vi "Width_Height to File Name.vi"(7 "include size in file name?":bool, 8 "keyword (\"\")":string, 10 "size":T1, 11 "VI file name (no extension)":string) -> (3 "file name":string)   [LabVIEW 2010, in "NI_SE_Front Panel Layout.lvlib"]
uses:
  NI_SE_Front Panel Layout.lvlib
  <vilib>/Utility/miscctls.llb/LVPointTypeDef.ctl
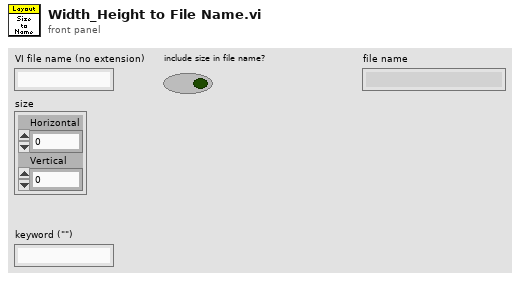
[diagram p1: front panel]
types:
  T1 = typedef "LVPointTypeDef.ctl" = cluster{"Horizontal":i16, "Vertical":i16}
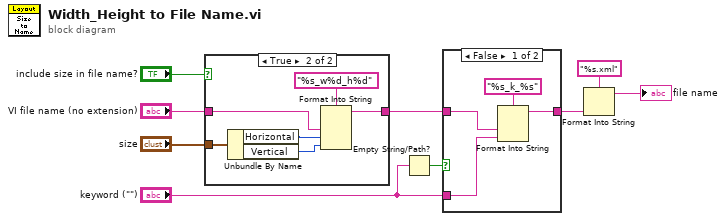
[diagram p0: block diagram]
diagram:
  n1 = case shown="True" "include size in file name?" {
    tunnel: "VI file name (no extension)" -> [w10 w15]
    tunnel: "size" -> [_ w13]
    tunnel: [w10 w14] -> w8
    frame False {
    }
    frame True {
      n2 = Unbundle By Name(w13) -> ("Horizontal"=w12:i16, "Vertical"=w11:i16)
      n3 = Format Into String(format string="%s_w%d_h%d", w15, w12, w11) -> (resulting string=w14:string)  [unwired: 2 in, 1 out]
    }
  }
  n4 = Empty String/Path?(string/path="keyword (\"\")") -> (empty?=w7:bool)
  n5 = case shown="False" w7 {
    tunnel: w8 -> [w19 w21]
    tunnel: "keyword (\"\")" -> [w17 _]
    tunnel: [w18 w21] -> w5
    frame False {
      n6 = Format Into String(format string="%s_k_%s", w19, w17) -> (resulting string=w18:string)  [unwired: 2 in, 1 out]
    }
    frame True {
    }
  }
  n7 = Format Into String(format string="%s.xml", w5) -> (resulting string=→"file name":string)  [unwired: 2 in, 1 out]
